vi "Set_Temp.vi"(7 "LS336FrontPanel.vi":bool, 8 "error in (no error)":errorcluster, 9 "Message_command_in":T1, 10 "Command_queue_in":T2) -> (0 "error out":errorcluster, 1 "Message_command_out":T1)   [LabVIEW 2025]
uses:
  Command_Message.ctl
  Command_Queue.ctl
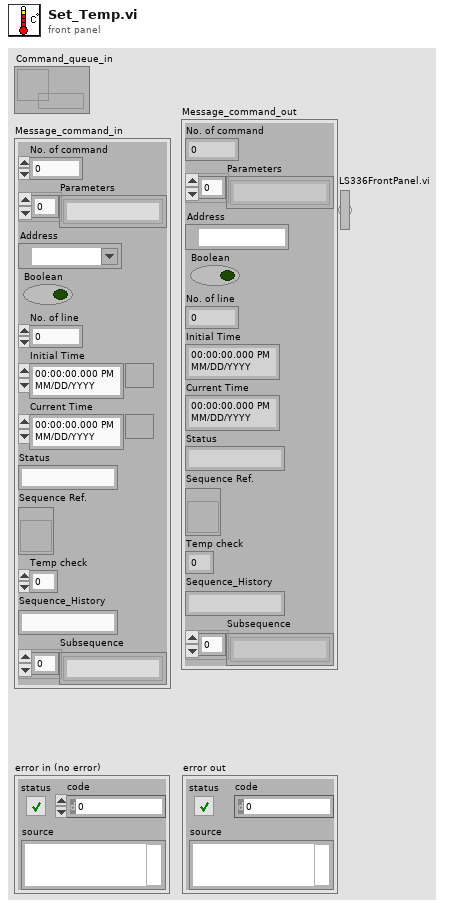
[diagram p1: front panel]
types:
  T1 = typedef "Command_Message.ctl" = cluster{"No. of command":i32, "Parameters":string[], "Address":refnum<visa-resource-name>, "Boolean":bool, "No. of line":i32, "Initial Time":timestamp, "Current Time":timestamp, "Status":string, "Sequence Ref.":refnum<vi>, "Temp check":i32, "Sequence_History":string, "Subsequence":string[]}
  T2 = typedef "Command_Queue.ctl" = refnum<queue>
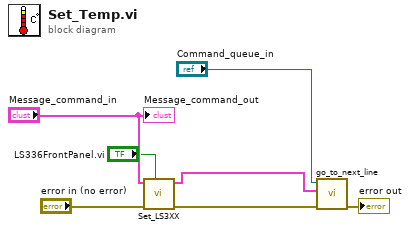
[diagram p0: block diagram]
diagram:
  n1 = call "Set_LS3XX.vi"("LS336FrontPanel.vi"="LS336FrontPanel.vi", "error in (no error)"="error in (no error)", "Message_command in"="Message_command_in") -> ("error out"=w1:errorcluster, "Message_command out"=w3:T1)  [unwired: 7 in]
  n2 = call "go_to_next_line.vi"("error in (no error)"=w1, "Message_command in"=w3, "Command Queue in"="Command_queue_in") -> ("error out"=→"error out":errorcluster)  [unwired: 7 in, 1 out]
  "Message_command_out" <- "Message_command_in"
